vi "ArcOpti_FGV.vi"(8 "error in":errorcluster, 10 "FGV_Control":u16(ring) items=["Set", "Get"], 11 "arcSet":bool=TRUE) -> (0 "error out":errorcluster, 3 "arcGet":bool)   [LabVIEW 2011]
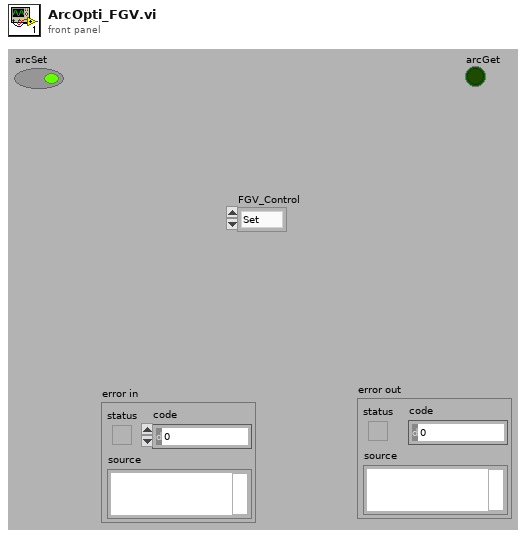
[diagram p1: front panel]
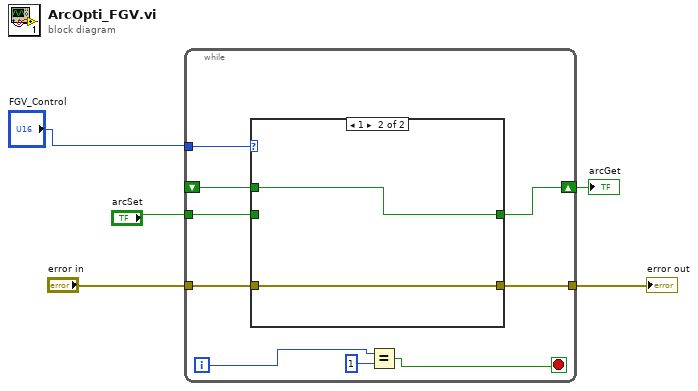
[diagram p0: block diagram]
diagram:
  n1 = while {
    tunnel: "FGV_Control" -> [w14]
    tunnel: "arcSet" -> [w13]
    shift-right: [w12] -> w4
    shift-left: _ -> [w11]
    tunnel: "error in" -> [w7]
    tunnel: [w6] -> w2
    i -> [w8]
    stop <- w9 stop-if-true
    n2 = case shown="1" w14 {
      tunnel: w13 -> [w16 _]
      tunnel: [w16 w18] -> w12
      tunnel: w11 -> [_ w18]
      tunnel: w7 -> [w15 w17]
      tunnel: [w15 w17] -> w6
      frame 0, Default {
      }
      frame 1 {
      }
    }
    n3 = Equal?(x=w8, y=1) -> (x = y?=w9:bool)
  }
  "arcGet" <- w4
  "error out" <- w2
